vi "Pre-Build Action.vi"(6 "Top Level/Always Included VIs":path[](array[path]) caption="Haupt-VIs/Immer enthaltene VIs", 7 "Main Destination Path":path caption="Hauptzielpfad", 9 "Target Name":string caption="Zielname", 10 "Build Specification Name":string caption="Name der Build-Spezifikation", 11 "Project Path":path caption="Projektpfad") -> (0 "error out":errorcluster caption="Fehler (Ausgang)")   [LabVIEW 2020]
uses:
  Projekteinstellungen/ConditionalDeactivation/ConditionalDeactivation.lvlib
  <vilib>/AppBuilder/AB_API_Simple/NI_App_Builder_API.lvlib
  <vilib>/AppBuilder/AB_API_Simple/Set Build Specification Version (path).vi
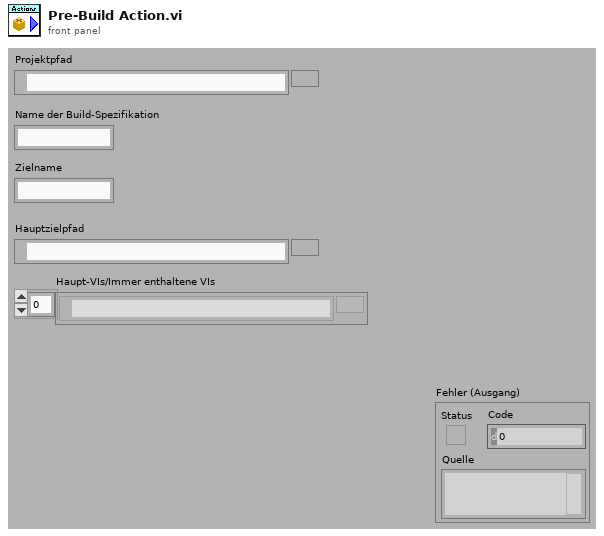
[diagram p1: front panel]
types:
  T1 = cluster{"Keys aus Projekt":string[], "Values aus Projekt":string[]}
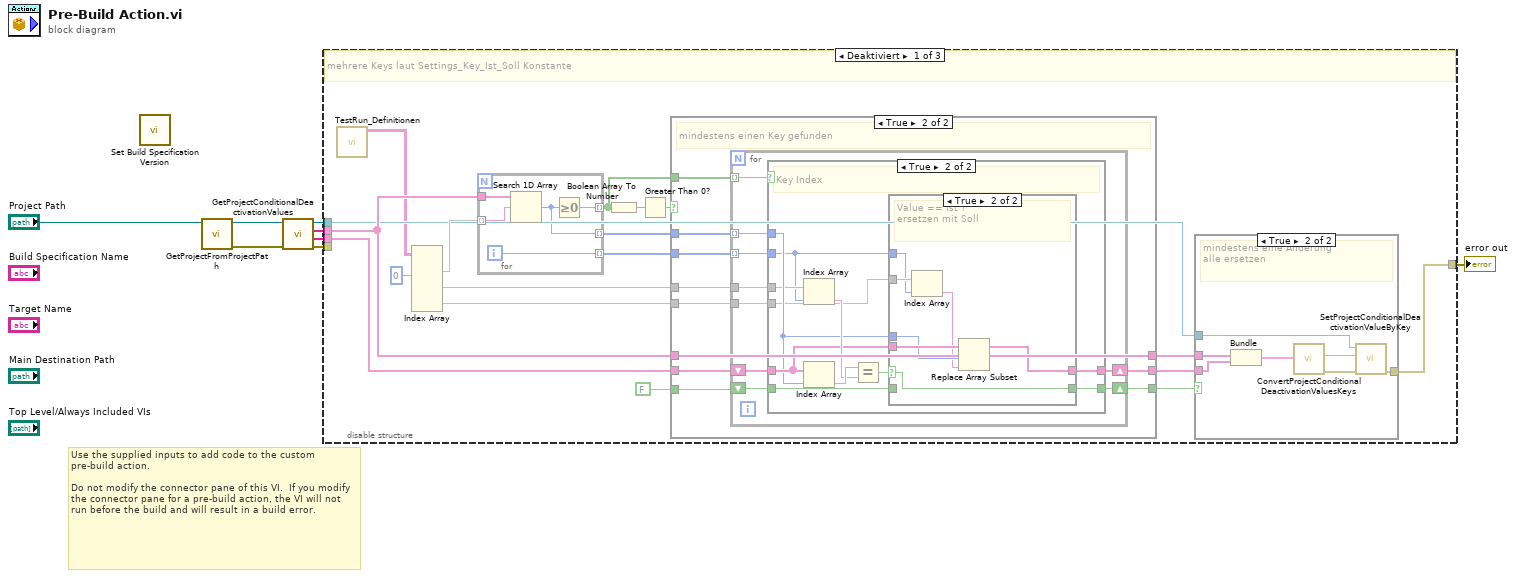
[diagram p0: block diagram]
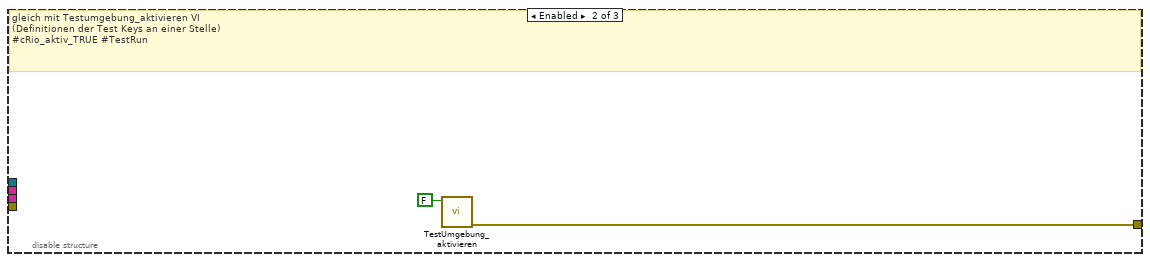
[diagram p6: hidden frame]
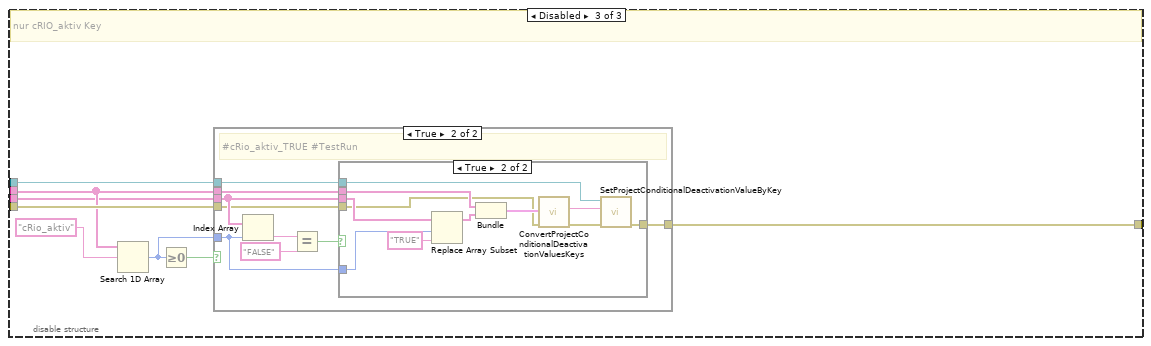
[diagram p7: hidden frame]
diagram:
  # "Use the supplied inputs to add code to the custom pre-build action.\n\nDo not modify the connector pane of this VI.  If you modify the connector pane for a pre-build action, the VI will not run before the build and will result in a build error."
  n1 = call-poly <vilib>:"Set Build Specification Version.vi"() -> ()  [unwired: 11 in, 1 out]
  n2 = call "GetProjectFromProjectPath.vi"("ProjectPfad"="Project Path") -> ("Fehler (Ausgang)"=w6:errorcluster, "Projekt Referenz"=w7:refnum<vi>)  [unwired: 9 in]
  n3 = call "GetProjectConditionalDeactivationValues.vi"("Fehler (Eingang, kein Fehler)"=w6, "Projekt Referenz"=w7) -> ("Fehler (Ausgang)"=w4:errorcluster, "Values aus Projekt"=w5:string[], "Keys aus Projekt"=w3:string[], "Projekt Referenz"=w1:refnum<vi>)  [unwired: 5 in, 1 out]
  n4 = disable-structure shown="Deaktiviert" {
    disable-tunnel: w3 -> [w21 _ w88]
    disable-tunnel: w5 -> [w20 _ w87]
    disable-tunnel: [w11 w83 w86] -> w2
    disable-tunnel: w4 -> [_ _ w90]
    disable-tunnel: w1 -> [w10 _ w85]
    frame Disabled {
      # "mehrere Keys laut Settings_Key_Ist_Soll Konstante"
      n5 = call "TestRun_Definitionen.vi"() -> ("Settings_Key_Ist_Soll"=w9:string[][])  [unwired: 11 in]
      n6 = Index Array(array=w9, index (col) #1=0 ("Deaktivierter Index (Spalte)")) -> (element #1=w26:string[], element #2=w18:string[], element #3=w17:string[])  [unwired: 5 in]
      n7 = for {
        tunnel: w26 -> [w81] mode=indexing
        tunnel: w21 -> [w82]
        tunnel: [w80] -> w22 mode=indexing
        tunnel: [w79] -> w23 mode=indexing
        tunnel: [w78] -> w16 mode=indexing
        i -> [w78]
        n8 = Search 1D Array(1D array=w82, element=w81) -> (index of element=w79:i32)  [unwired: 1 in]
        n9 = Greater Or Equal To 0?(x=w79) -> (x >= 0?=w80:bool)
      }
      n10 = Boolean Array To Number(Boolean array=w22) -> (number=w25:u32)
      n11 = Greater Than 0?(x=w25) -> (x > 0?=w24:bool)
      n12 = case shown="True" w24 {
        tunnel: w23 -> [_ w45]
        tunnel: w22 -> [_ w46]
        tunnel: w21 -> [w35 w39]
        tunnel: w20 -> [w36 w44]
        tunnel: w18 -> [_ w42]
        tunnel: w17 -> [_ w41]
        tunnel: w16 -> [_ w43]
        tunnel: [w36 w40] -> w12
        tunnel: [w35 w39] -> w13
        tunnel: [w34 w38] -> w14
        tunnel: FALSE -> [w34 w37]
        frame False {
        }
        frame True {
          # "mindestens einen Key gefunden"
          n13 = for {
            tunnel: w46 -> [w55] mode=indexing
            tunnel: w45 -> [w53] mode=indexing
            tunnel: w43 -> [w52] mode=indexing
            tunnel: w42 -> [w51]
            tunnel: w41 -> [w50]
            shift-right: [w49] -> w40
            shift-left: w44 -> [w54]
            shift-right: [w48] -> w38
            shift-left: w37 -> [w47]
            n14 = case shown="True" w55 {
              tunnel: w54 -> [w57 w65]
              tunnel: w53 -> [_ w64]
              tunnel: w52 -> [_ w61]
              tunnel: w51 -> [_ w63]
              tunnel: w50 -> [_ w62]
              tunnel: [w57 w60] -> w49
              tunnel: [w56 w59] -> w48
              tunnel: w47 -> [w56 w58]
              frame False {
              }
              frame True {
                # "Key Index"
                n15 = Index Array(array=w63, index=w61) -> (element=w67:string)
                n16 = Index Array(array=w65, index=w64) -> (element=w68:string)
                n17 = Equal?(x=w68, y=w67) -> (x = y?=w66:bool)
                n18 = case shown="True" w66 {
                  selector: w66 -> [_ w71]
                  tunnel: w65 -> [w70 w77]
                  tunnel: w64 -> [_ w76]
                  tunnel: w62 -> [_ w75]
                  tunnel: w61 -> [_ w74]
                  tunnel: [w70 w72] -> w60
                  tunnel: [w69 w71] -> w59
                  tunnel: w58 -> [w69 _]
                  frame False {
                  }
                  frame True {
                    # "Value == Ist ?\nersetzen mit Soll"
                    n19 = Index Array(array=w75, index=w74) -> (element=w73:string)
                    n20 = Replace Array Subset(array=w77, new element=w73, index=w76) -> (w72:string[])
                  }
                }
              }
            }
          }
        }
      }
      n21 = case shown="True" w14 {
        tunnel: w13 -> [_ w30]
        tunnel: w12 -> [_ w29]
        tunnel: [_ w28] -> w11
        tunnel: w10 -> [_ w27]
        frame False {
        }
        frame True {
          # "mindestens eine Änderung\nalle ersetzen"
          n22 = Bundle("Keys aus Projekt"=w30, "Values aus Projekt"=w29) -> (w31:T1)  [unwired: 1 in]
          n23 = call "ConvertProjectConditionalDeactivationValuesKeys.vi"("CondDeact"=w31) -> ("Fehler (Ausgang)"=w32:errorcluster, "Tabellen-String"=w33:string)  [unwired: 9 in]
          n24 = call "SetProjectConditionalDeactivationValueByKey.vi"("Fehler (Eingang, kein Fehler)"=w32, "Tabellen-String"=w33, "Projekt Referenz"=w27) -> ("Fehler (Ausgang)"=w28:errorcluster)  [unwired: 7 in, 1 out]
        }
      }
    }
    frame Enabled {
      # "gleich mit Testumgebung_aktivieren VI  \n(Definitionen der Test Keys an einer Stelle)\n#cRio_aktiv_TRUE #TestRun"
      n25 = call "TestUmgebung_aktivieren.vi"("TestUmgebung aktiv/inaktiv"=FALSE) -> ("Fehler (Ausgang)"=w83:errorcluster)  [unwired: 10 in]
    }
    frame Disabled {
      # "nur cRIO_aktiv Key"
      n26 = Search 1D Array(1D array=w88, element="cRio_aktiv") -> (index of element=w92:i32)  [unwired: 1 in]
      n27 = Greater Or Equal To 0?(x=w92) -> (x >= 0?=w91:bool)
      n28 = case shown="True" w91 {
        tunnel: w88 -> [_ w98]
        tunnel: w87 -> [_ w97]
        tunnel: w92 -> [_ w96]
        tunnel: [_ w95] -> w86
        tunnel: w90 -> [_ w94]
        tunnel: w85 -> [_ w93]
        frame False {
        }
        frame True {
          # "#cRio_aktiv_TRUE #TestRun"
          n29 = Index Array(array=w97, index=w96) -> (element=w101:string)
          n30 = Equal?(x=w101, y="FALSE") -> (x = y?=w99:bool)
          n31 = case shown="True" w99 {
            tunnel: w98 -> [_ w105]
            tunnel: w97 -> [_ w112]
            tunnel: w96 -> [_ w111]
            tunnel: [_ w104] -> w95
            tunnel: w94 -> [_ w103]
            tunnel: w93 -> [_ w102]
            frame False {
            }
            frame True {
              n32 = Replace Array Subset(array=w112, new element="TRUE" ("Neues Element/Teil-Array"), index=w111) -> (w106:string[])
              n33 = Bundle("Keys aus Projekt"=w105, "Values aus Projekt"=w106) -> (w107:T1)  [unwired: 1 in]
              n34 = call "ConvertProjectConditionalDeactivationValuesKeys.vi"("Fehler (Eingang, kein Fehler)"=w103, "CondDeact"=w107) -> ("Fehler (Ausgang)"=w108:errorcluster, "Tabellen-String"=w109:string)  [unwired: 8 in]
              n35 = call "SetProjectConditionalDeactivationValueByKey.vi"("Fehler (Eingang, kein Fehler)"=w108, "Tabellen-String"=w109, "Projekt Referenz"=w102) -> ("Fehler (Ausgang)"=w104:errorcluster)  [unwired: 7 in, 1 out]
            }
          }
        }
      }
    }
  }
  "error out" <- w2
